vi "turret_degrees_to_raw.vi"(10 "Degrees In":dbl) -> (2 "Raw Encoder Units Out":dbl)   [LabVIEW 2020]
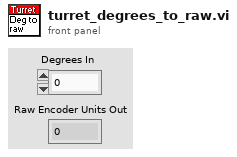
[diagram p1: front panel]
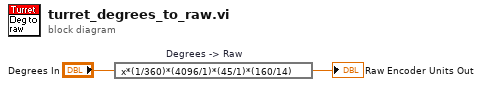
[diagram p0: block diagram]
diagram:
  n1 = expression code="x*(1/360)*(4096/1)*(45/1)*(160/14)" "Degrees -> Raw"("Degrees In") -> (→"Raw Encoder Units Out":dbl)
